vi "Counter - Continuous Output.vi"() -> ()   [LabVIEW 2012]
doc: "This example demonstrates how to continuously generate digital pulses using a counter output."
uses:
  <vilib>/DAQmx/create/channels.llb/DAQmx Create Channel (CO-Pulse Generation-Frequency).vi
  <vilib>/DAQmx/configure/timing.llb/DAQmx Timing (Implicit).vi
  <vilib>/DAQmx/configure/trigger.llb/DAQmx Start Trigger (Digital Edge).vi
  <resource>/objmgr/daqmx.rc
panel:
  in  "CO.Pulse.DutyCyc":dbl(slide)=0.01 min=0.01 max=0.99 step=0.1 scale=0.0..1.0
  out "Actual Duty Cycle":dbl
  out "Actual Frequency":dbl
  in  "Duty Cycle":dbl=0.5 format="%.6f"
  in  "Frequency":dbl=1.0 format="%.6f"
  in  "Output Terminal":tag="/Dev1/PFI12"
  in  "Trigger Type":T1(tab)
  in  "Edge":i32(ring)=10280 items=["Rising"=10280, "Falling"=10171]
  in  "Digital Trigger Source":tag
  in  "Pause When":i32(ring)=10192 items=["High"=10192, "Low"=10214]
  in  "Pause Trigger Source":tag
  in  "Stop":bool
  in  "Counter":tag="Dev1/ctr0"
  # "Channel Settings"
  # "Trigger Settings"
  # "To configure and use a trigger you must have the necessary tab selected above."
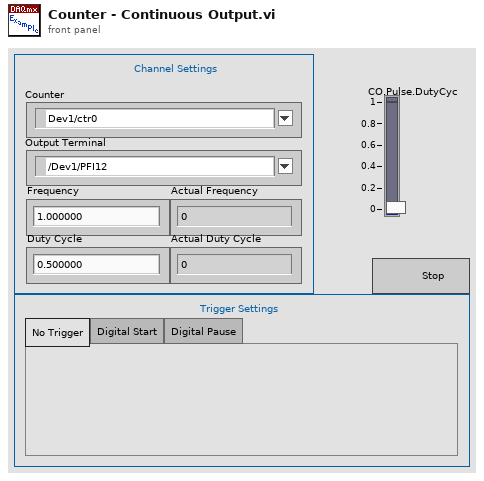
[diagram p1: front panel]
types:
  T1 = enum32{"No Trigger", "Digital Start", "Digital Pause"}
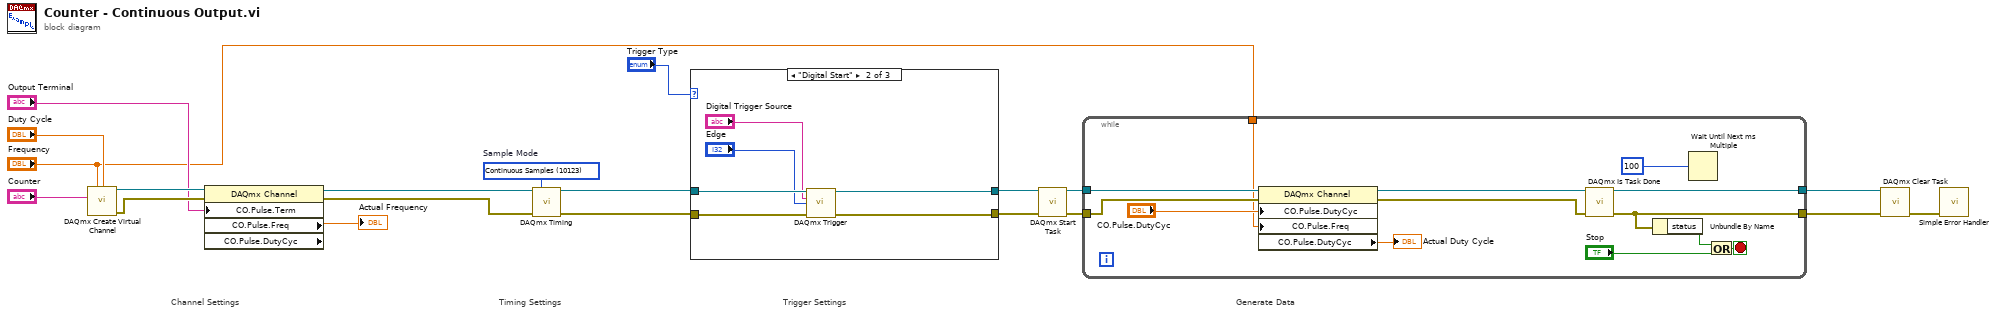
[diagram p0: block diagram]
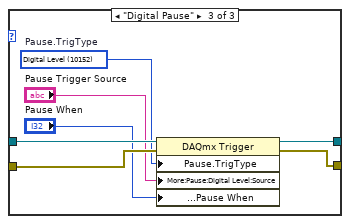
[diagram p3: hidden frame]
diagram:
  w20 = 10123 items=["Finite Samples"=10178, "Continuous Samples"=10123, "Hardware Timed Single Point"=12522]  # Sample Mode
  # "Generate Data"
  # "Trigger Settings"
  # "Timing Settings"
  # "Channel Settings"
  n1 = call-poly <vilib>:"DAQmx Create Virtual Channel.vi"("frequency"="Frequency", "duty cycle"="Duty Cycle", "counter"="Counter") -> ("task out"=w8:refnum<k21>, "error out"=w7:errorcluster)  [unwired: 11 in]
  n2 = property class="DAQmx Channel" props=["CO.Pulse.Term", "CO.Pulse.Freq", "CO.Pulse.DutyCyc"](reference=w8, error in=w7, "CO.Pulse.Term"="Output Terminal") -> (reference out=w4:refnum<k21>, error out=w5:errorcluster, "CO.Pulse.Freq"=→"Actual Frequency":dbl)  [unwired: 1 out]
  n3 = call-poly <vilib>:"DAQmx Timing.vi"("task/channels in"=w4, "sample mode"=w20, "error in"=w5) -> ("task out"=w12:refnum<k21>, "error out"=w11:errorcluster)  [unwired: 11 in]
  n4 = case shown="\"Digital Start\"" "Trigger Type" {
    tunnel: w12 -> [w22 w28 w35]
    tunnel: w11 -> [w21 w27 w32]
    tunnel: [w22 w26 w34] -> w9
    tunnel: [w21 w25 w33] -> w10
    frame "No Trigger", Default {
    }
    frame "Digital Start" {
      n5 = call-poly <vilib>:"DAQmx Trigger.vi"("task/channels in"=w28, "source"="Digital Trigger Source", "edge"="Edge", "error in"=w27) -> ("task out"=w26:refnum<k21>, "error out"=w25:errorcluster)  [unwired: 10 in]
    }
    frame "Digital Pause" {
      w31 = 10152 items=["Analog Level"=10101, "Analog Window"=10103, "Digital Level"=10152, "Digital Pattern"=10398, "None"=10230]  # Pause.TrigType
      n6 = property class="DAQmx Trigger"(reference=w35, error in=w32, "Pause.TrigType"=w31, "More:Pause:Digital Level:Source"="Pause Trigger Source", "More:Pause:Digital Level:Pause When"="Pause When") -> (reference out=w34:refnum<k21>, error out=w33:errorcluster)
    }
  }
  n7 = call <vilib>:"DAQmx Start Task.vi"("task/channels in"=w9, "error in"=w10) -> ("task out"=w19:refnum<k21>, "error out"=w18:errorcluster)  [unwired: 12 in]
  n8 = while {
    tunnel: w19 -> [w42]
    tunnel: w18 -> [w39]
    tunnel: [w46] -> w16
    tunnel: [w47] -> w17
    tunnel: "Frequency" -> [w36]
    stop <- w48 stop-if-true
    n9 = property class="DAQmx Channel"(reference=w42, error in=w39, "CO.Pulse.DutyCyc"="CO.Pulse.DutyCyc", "CO.Pulse.Freq"=w36) -> (reference out=w41:refnum<k21>, error out=w38:errorcluster, "CO.Pulse.DutyCyc"=→"Actual Duty Cycle":dbl)
    n10 = call <vilib>:"DAQmx Is Task Done.vi"("task/channels in"=w41, "error in"=w38) -> ("task out"=w47:refnum<k21>, "error out"=w46:errorcluster)  [unwired: 11 in, 1 out]
    n11 = Unbundle By Name(w46) -> ("status"=w45:bool)
    n12 = Wait Until Next ms Multiple(millisecond multiple=u32 100) -> ()  [unwired: 1 out]
    n13 = Or(x=w45, y="Stop") -> (x .or. y?=w48:bool)
  }
  n14 = call <vilib>:"DAQmx Clear Task.vi"("task in"=w17, "error in"=w16) -> ("error out"=w15:errorcluster)  [unwired: 13 in]
  n15 = call <vilib>:"Simple Error Handler.vi"("error in (no error)"=w15) -> ()  [unwired: 4 in, 5 out]
